vi "ASI Stage.vi"() -> (3 "VISA resource name out":refnum<visa-resource-name>)   [LabVIEW 2012]
uses:
  <vilib>/Instr/_visa.llb/VISA Configure Serial Port (Instr).vi
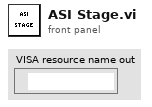
[diagram p1: front panel]
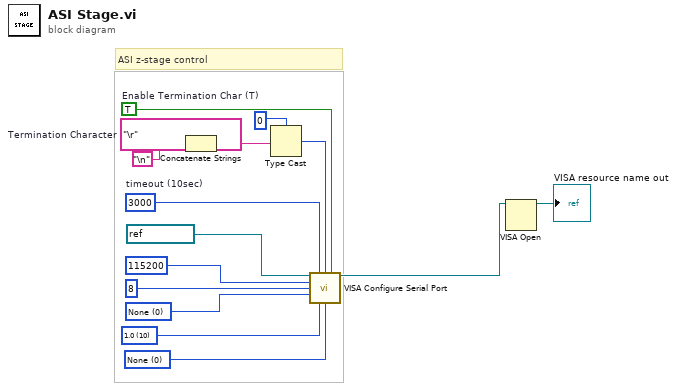
[diagram p0: block diagram]
diagram:
  w12 = u16 0 items=["None"=0, "XON/XOFF"=1, "RTS/CTS"=2, "DTR/DSR"=4] ("flow control")
  w11 = u16 10 items=["1.0"=10, "1.5"=15, "2.0"=20] ("stop bits")
  w8 = u16 0 items=["None", "Odd", "Even", "Mark", "Space"] ("parity")
  w5 = "\r"  # Termination Character
  w10 = TRUE  # Enable Termination Char (T)
  w9 = u32 3000  # timeout (10sec)
  # "ASI z-stage control"
  n1 = Concatenate Strings(w5, "\n") -> (w3:string)
  n2 = Type Cast(type=u8 0, x=w3) -> (*(type *) &x=w15:u8)
  n3 = call-poly "VISA Configure Serial Port"("VISA resource name"=refnum<visa-resource-name> "COM17" ("COM17"), "timeout (10sec)"=w9, "termination char\n(0xA = '\\n' = LF)"=w15, "Enable Termination\nChar (T)"=w10, "baud rate (9600)"=u32 115200 ("baud rate"), "data bits (8)"=u16 8 ("data bits"), "parity (0:none)"=w8, "stop bits (10: 1 bit)"=w11, "flow control (0:none)"=w12) -> ("VISA resource name out"=w2:refnum<visa-resource-name>)  [unwired: 5 in, 1 out]
  n4 = VISA Open(VISA resource name=w2) -> (VISA resource name=→"VISA resource name out":refnum<visa-resource-name>)  [unwired: 4 in, 1 out]
